vi "Pressure_Multiplexer_Server2.vi"(4 "DAQ Tigger Control?":bool, 6 "DAQ Trigger Port":refnum<visa-resource-name>="COM100", 7 "Analysis Info cluster":T4[](array[typedef]) {"Sync Delay Time (s)" format="%.4f"; "Total Meas Time (s)" format="%_5g"; "Sd Error in Variance" format="%_3g"; "Skew_u" format="%_3g"; "% u'/U" format="%_3g"; "Sd Error in Mean" format="%_3g"; "Kurt_u" format="%_3g"; "u^4" format="%_3g"; "u^3" format="%_3g"; "U" format="%_3g"; "u^2" format="%_3g"}, 8 "Current Block No":i32, 9 "Time per Block (s)":dbl=100.0 format="%_4f", 10 "setup":T3=enum."Show Setup", 11 "Trigger mode":T2) -> (0 "DAQ Error":errorcluster, 2 "Index with data":i32[](array[numeric]), 3 "Time Trace":T1[](array[typedef]))   [LabVIEW 2022 SP3]
uses:
  Controls/Analysis_info_cluster.ctl
  Controls/Inst_type.ctl
  Controls/Instrument_Array.ctl
  Controls/Setup.ctl
  Controls/Trigger_Mode.ctl
  Controls/Time_Trace_Cluster.ctl
  Globals/Meas_global.vi
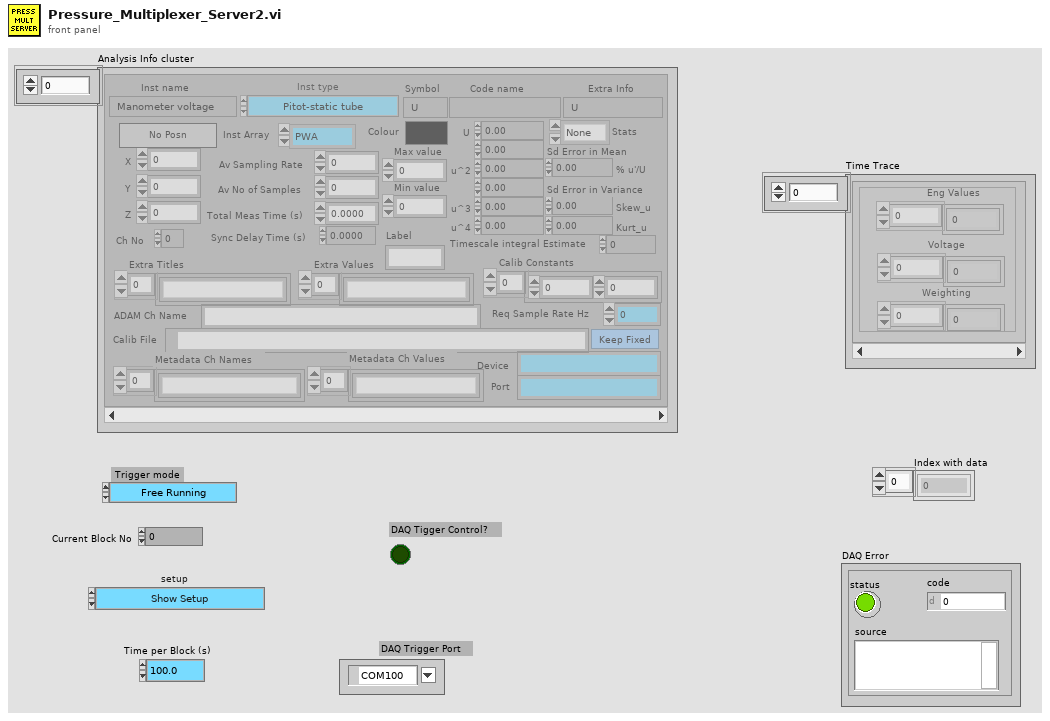
[diagram p1: front panel]
types:
  T1 = typedef "Time_Trace_Cluster.ctl" = cluster{"Weighting":dbl[], "Voltage":dbl[], "Eng Values":dbl[]}
  T2 = typedef "Trigger_Mode.ctl" = enum16{"Free Running", "Start on Trigger", "Trigger Every Block", "Trigger Every Sample"}
  T3 = typedef "Setup.ctl" = enum16{"Run Program", "Show Setup", "Save Current Setup", "Setup Front Panel"}
  T4 = typedef "Analysis_info_cluster.ctl" = cluster{"Colour":u32, "Inst type":T5, "Inst name":string, "Symbol":string, "Code name":string, "Extra Info":string, "Inst Array":T6, "Extra Titles":string[], "Extra Values":string[], "U":dbl, "u^2":dbl, "u^3":dbl, "u^4":dbl, "Skew_u":dbl, "Kurt_u":dbl, "Sd Error in Mean":dbl, "% u'/U":dbl, "X":dbl, "Y":dbl, "Z":dbl, "Timescale integral Estimate":dbl, "Sd Error in Variance":dbl, "Calib File":path, "Calib Constants":dbl[], "Output Position":bool, "Stats":enum16{"None", "Basic", "Full"}, "Av Sampling Rate":dbl, "Av No of Samples":dbl, "Total Meas Time (s)":dbl, "ADAM Ch Name":string, "Max value":dbl, "Min value":dbl, "Req Sample Rate Hz":dbl, "Sync Delay Time (s)":dbl, "Ch No":i16, "Device":string, "Use Latest Calib":bool, "Port":string, "Metadata Ch Names":string[], "Metadata Ch Values":string[], "Label":string}
  T5 = typedef "Inst_type.ctl" = enum16{"Raw voltage", "Raw with zero offsetting", "Propeller anemometer", "Pressure Transducer", "Pitot-static tube", "Hot wire", "Cross wire 1", "Cross wire 2", "Generic Linear", "Generic Polynomial", "Generic BackPoly", "Fast FID", "Thermocouple", "Cold wire", "Pulsed Wire", "LDA Vel", "LDA Tran time", "LDA Arr time", "Microphone"}
  T6 = typedef "Instrument_Array.ctl" = enum16{"PWA", "LDA", "Analogue"}
  T7 = typedef "Device ID port info.ctl" = cluster{"Ch No":i16[], "Req Sampling Rate":dbl[], "Port":string, "Index":i32[]}
  T8 = typedef "Rendezvous RefNum" = refnum<k1>
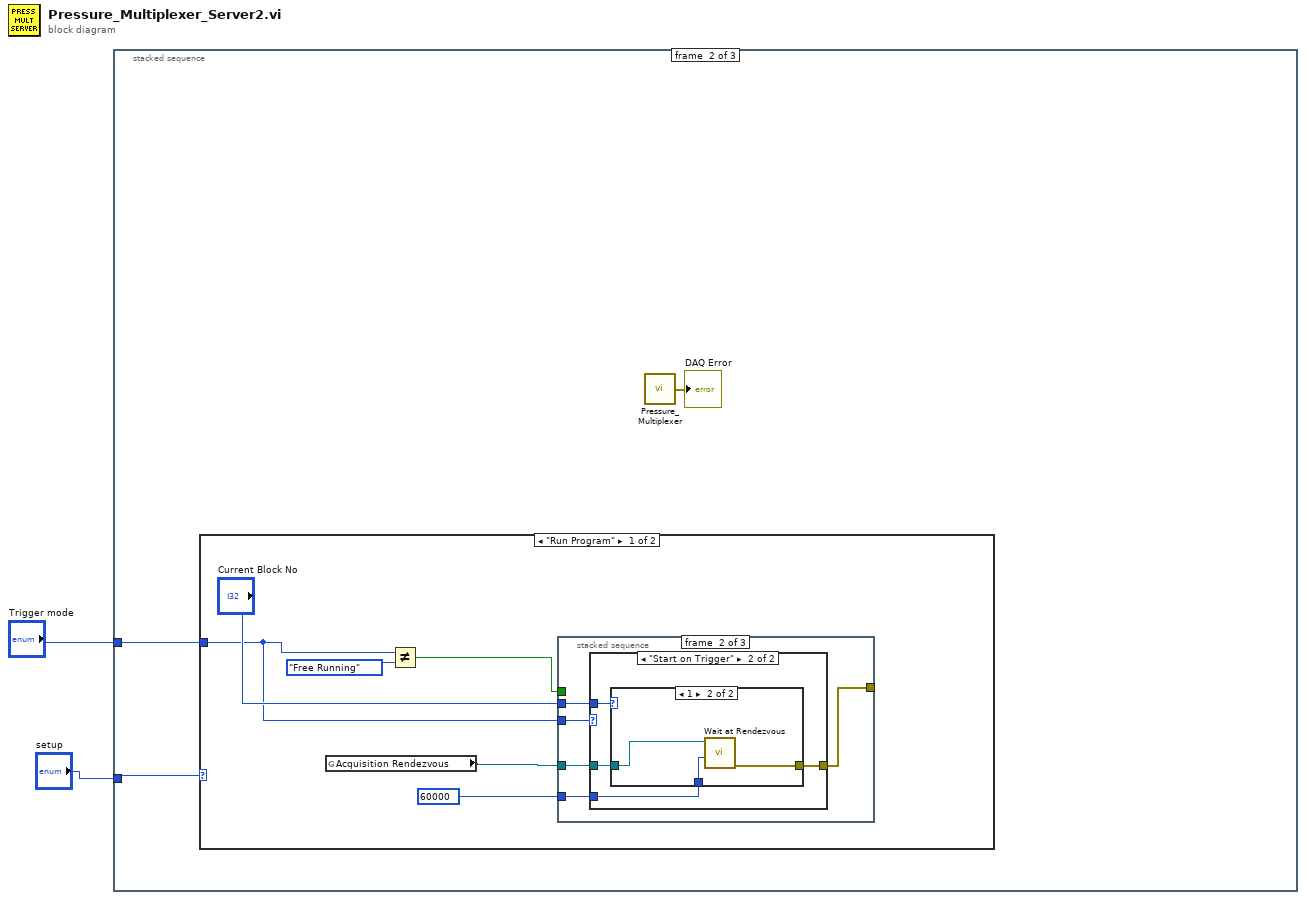
[diagram p0: block diagram]
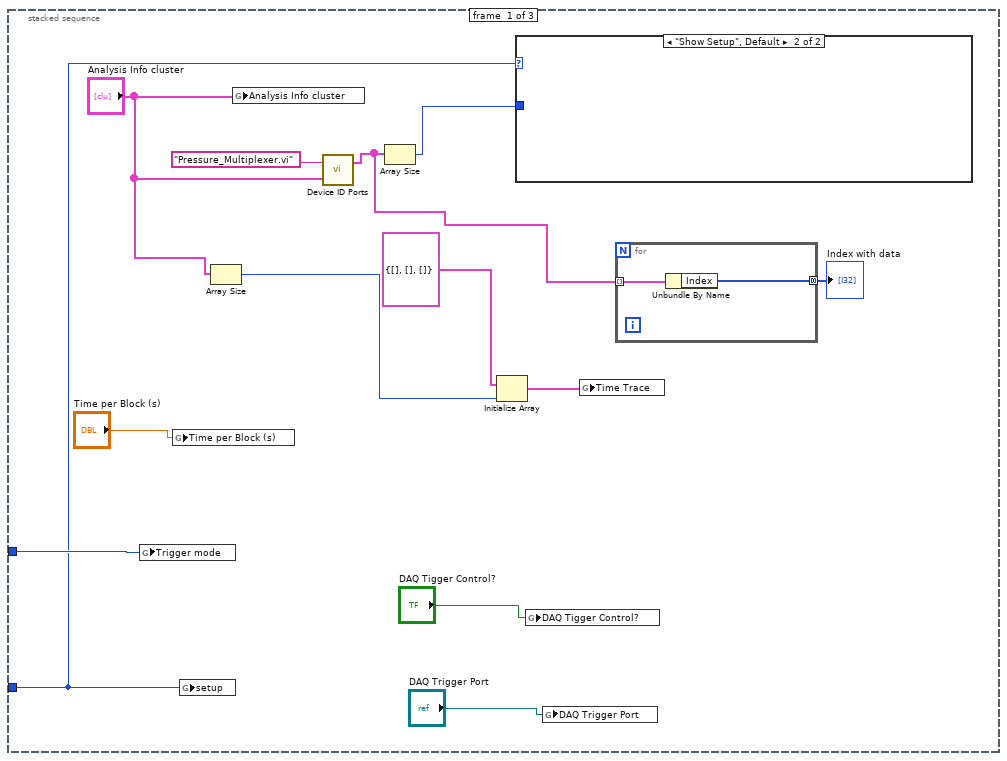
[diagram p2: hidden frame]
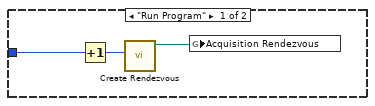
[diagram p3: hidden frame]
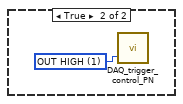
[diagram p5: hidden frame]
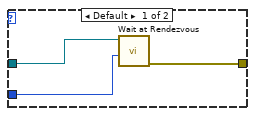
[diagram p6: hidden frame]
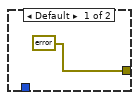
[diagram p7: hidden frame]
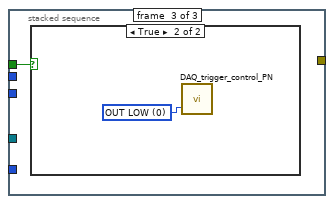
[diagram p8: hidden frame]
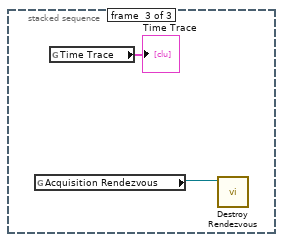
[diagram p11: hidden frame]
diagram:
  n1 = stacked-sequence {
    tunnel: "Trigger mode" -> [w10 w23 _]
    tunnel: "setup" -> [w3 w21 _]
    frame #0 {
      n2 = global write "Meas_global.vi" "Trigger mode"(w10) -> ()
      n3 = global write "Meas_global.vi" "Time per Block (s)"("Time per Block (s)") -> ()
      n4 = global write "Meas_global.vi" "setup"(w3) -> ()
      n5 = Array Size(array="Analysis Info cluster") -> (size(s)=w7:i32)
      n6 = global write "Meas_global.vi" "Analysis Info cluster"("Analysis Info cluster") -> ()
      n7 = call "Device ID Ports.vi"("Analysis Info cluster"="Analysis Info cluster", "Device ID"="Pressure_Multiplexer.vi") -> ("Device port info"=w5:T7[])  [unwired: 1 out]
      n8 = Array Size(array=w5) -> (size(s)=w11:i32)
      n9 = Initialize Array(T1 {"Weighting"=[], "Voltage"=[], "Eng Values"=[]} ("element"), w7) -> (w6:T1[])
      n10 = case shown="\"Show Setup\", Default" w3 {
        tunnel: w11 -> [w17 _]
        frame "Run Program" {
          n11 = Increment(x=w17) -> (x+1=w18:i32)
          n12 = call <vilib>:"Create Rendezvous.vi"("size (2)"=w18) -> ("rendezvous"=w16:T8)  [unwired: 4 in, 2 out]
          n13 = global write "Meas_global.vi" "Acquisition Rendezvous"(w16) -> ()
        }
        frame "Show Setup", Default {
        }
      }
      n14 = global write "Meas_global.vi" "DAQ Tigger Control?"("DAQ Tigger Control?") -> ()
      n15 = global write "Meas_global.vi" "DAQ Trigger Port"("DAQ Trigger Port") -> ()
      n16 = global write "Meas_global.vi" "Time Trace"(w6) -> ()
      n17 = for {
        tunnel: w5 -> [w20] mode=indexing
        tunnel: [w19] -> w4 mode=concatenating
        n18 = Unbundle By Name(w20) -> ("Index"=w19:i32[])
      }
      "Index with data" <- w4
    }
    frame #1 {
      n19 = case shown="\"Run Program\"" w21 {
        tunnel: w23 -> [w25 _]
        frame "Run Program" {
          n20 = global read "Meas_global.vi" "Acquisition Rendezvous"() -> (w24:T8)
          n21 = Not Equal?(x=w25, y=Trigger_Mode."Free Running" ("Trigger mode")) -> (x != y?=w28:bool)
          n22 = stacked-sequence {
            tunnel: [_ w35 _] -> _
            tunnel: w28 -> [w30 _ w48]
            tunnel: "Current Block No" -> [_ w36 _]
            tunnel: w25 -> [_ w34 _]
            tunnel: 60000 ("ms timeout (-1)") -> [_ w33 _]
            tunnel: w24 -> [_ w32 _]
            frame #0 {
              n23 = case shown="False" w30 {
                frame False {
                }
                frame True {
                  w31 = u8 1 items=["OUT LOW", "OUT HIGH", "IN READ"] ("Action")
                  n24 = call "DAQ_trigger_control_PN.vi"("Action"=w31) -> ()  [unwired: 1 in, 3 out]
                }
              }
            }
            frame #1 {
              n25 = case shown="\"Start on Trigger\"" w34 {
                tunnel: w36 -> [_ w43]
                tunnel: [w39 w42] -> w35
                tunnel: w33 -> [w38 w41]
                tunnel: w32 -> [w37 w40]
                frame Default {
                  n26 = call <vilib>:"Wait at Rendezvous.vi"("ms timeout (-1)"=w38, "rendezvous"=w37) -> ("error out"=w39:errorcluster)  [unwired: 3 in, 2 out]
                }
                frame "Start on Trigger" {
                  n27 = case shown="1" w43 {
                    tunnel: [errorcluster {"status"=FALSE, "code"=0, "source"=""} ("error out") w47] -> w42
                    tunnel: w41 -> [_ w46]
                    tunnel: w40 -> [_ w45]
                    frame Default {
                    }
                    frame 1 {
                      n28 = call <vilib>:"Wait at Rendezvous.vi"("ms timeout (-1)"=w46, "rendezvous"=w45) -> ("error out"=w47:errorcluster)  [unwired: 3 in, 2 out]
                    }
                  }
                }
              }
            }
            frame #2 {
              n29 = case shown="True" w48 {
                frame False {
                }
                frame True {
                  w49 = u8 0 items=["OUT LOW", "OUT HIGH", "IN READ"] ("Action")
                  n30 = call "DAQ_trigger_control_PN.vi"("Action"=w49) -> ()  [unwired: 1 in, 3 out]
                }
              }
            }
          }
        }
        frame "Show Setup", Default {
        }
      }
      n31 = call "Pressure_Multiplexer.vi"() -> ("DAQ Error"=→"DAQ Error":errorcluster)  [unwired: 1 in]
    }
    frame #2 {
      n32 = global read "Meas_global.vi" "Acquisition Rendezvous"() -> (w51:T8)
      n33 = global read "Meas_global.vi" "Time Trace"() -> (→"Time Trace":T1[])
      n34 = call <vilib>:"Destroy Rendezvous.vi"("rendezvous"=w51) -> ()  [unwired: 5 in, 2 out]
    }
  }
